vi "Switch Subpanel.vi"(8 "error in (no error)":errorcluster, 10 "Subpanel Type":T1, 11 "CIF_UI in":refnum<class "CIF_UI.lvclass">) -> (0 "error out":errorcluster, 2 "VI Reference":refnum<vi>, 3 "CIF_UI out":refnum<class "CIF_UI.lvclass">)   [LabVIEW 2021, in "CIF_UI.lvclass"]
uses:
  CIF_UI.lvclass
  Typedef/Subpanel Type.ctl
  CIF_UI.lvclass/CIF_UI.ctl
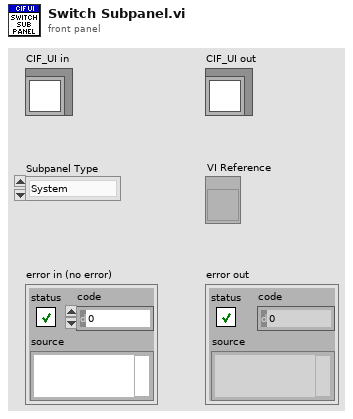
[diagram p1: front panel]
types:
  T1 = typedef "CIF_UI.lvclass/Subpanel Type.ctl" = enum16{"System", "Errors", "Channel", "Plugin"}
  T2 = typedef "CIF_UI.lvclass/Subpanel Map.ctl" = map{T1, T3}
  T3 = typedef "CIF_UI.lvclass/Subpanel Data.ctl" = cluster{"VI Reference":refnum<vi>}
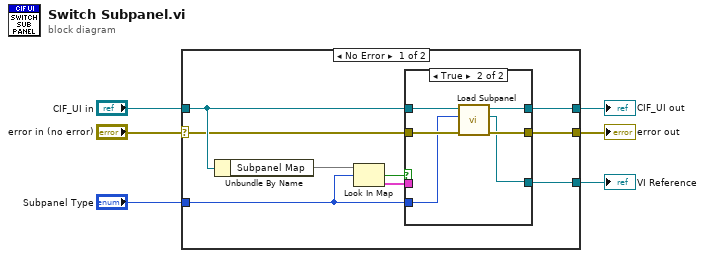
[diagram p0: block diagram]
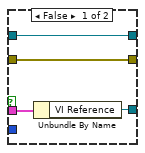
[diagram p2: hidden frame]
diagram:
  n1 = case shown="No Error" "error in (no error)" {
    selector: "error in (no error)" -> [w9 w27]
    tunnel: [w8 w27] -> w5
    tunnel: [w10 w26] -> w3
    tunnel: "CIF_UI in" -> [w12 w26]
    tunnel: "Subpanel Type" -> [w11 _]
    tunnel: [w7 _] -> w1
    frame No Error {
      n2 = Unbundle By Name(w12) -> ("Subpanel Map"=w15:T2)
      n3 = Look In Map(map=w15, key=w11) -> (key not found?=w14:bool, value=w13:T3)  [unwired: 1 in]
      n4 = case shown="True" w14 {
        tunnel: w13 -> [w19 _]
        tunnel: w12 -> [w18 w25]
        tunnel: w11 -> [_ w22]
        tunnel: [w18 w24] -> w10
        tunnel: w9 -> [w17 w23]
        tunnel: [w17 w21] -> w8
        tunnel: [w16 w20] -> w7
        frame False {
          n5 = Unbundle By Name(w19) -> ("VI Reference"=w16:refnum<vi>)
        }
        frame True {
          n6 = call "Load Subpanel.vi"("error in (no error)"=w23, "Subpanel Type"=w22, "CIF_UI in"=w25) -> ("error out"=w21:errorcluster, "VI Reference"=w20:refnum<vi>, "CIF_UI out"=w24:refnum<class "CIF_UI.lvclass">)  [unwired: 6 in]
        }
      }
    }
    frame Error {
    }
  }
  "error out" <- w5
  "CIF_UI out" <- w3
  "VI Reference" <- w1
